vi "Tatrocki_B_1.vi"   [LabVIEW 2020]
uses:
  <vilib>/Platform/TimedLoop/XDataNode/timing_clust.ctl
  <vilib>/Platform/TimedLoop/XDataNode/nitl_modes.ctl
  <vilib>/Platform/TimedLoop/XDataNode/wakeup.ctl
  <vilib>/platform/TimedLoop/XDataNode/XDataNode.xnode
  <vilib>/Platform/TimedLoop/XDataNode/XDNodeRunTimeDep.lvlib
types:
  T1 = typedef "Rendezvous RefNum" = refnum<k1>
  T2 = typedef "Semaphore RefNum" = refnum<k1>
  T3 = typedef "XDNodeRunTimeDep.lvlib/timing_clust.ctl" = cluster{"Expected End [f-1]":u64, "Actual End [f-1]":u64, "Finished Late? [f-1]":bool, "Expected End [i-1]":u64, "Actual End [i-1]":u64, "Finished Late? [i-1]":bool, "Expected Start [i]":u64, "Actual Start [i]":u64, "Expected Start [f]":u64, "Actual Start [f]":u64, "Source Name":string, "Structure Name":string, "Period":i64, "Deadline":i64, "Offset":i64, "Start":i64, "Priority":i32, "Timeout":i32, "Mode":T4, "Wakeup Reason":T5, "Error":errorcluster, "Source Type":string, "Secondary Source Type":string, "Global End Time":u64, "Global Start Time":u64, "Frame Duration":u64, "Iteration Duration":u64, "Assigned CPU":i32, "I/O Scan Engine Mode":u32}
  T4 = typedef "XDNodeRunTimeDep.lvlib/nitl_modes.ctl" = enum32{"No Change", "Process missed periods, maintain original phase", "Discard missed periods, maintain original phase", "Process missed periods, ignore original phase", "Discard missed periods, ignore original phase"}
  T5 = typedef "XDNodeRunTimeDep.lvlib/wakeup.ctl" = enum32{"Normal", "Aborted", "Asynchronous wakeup", "Timing source error", "Timed loop error", "Timeout"}
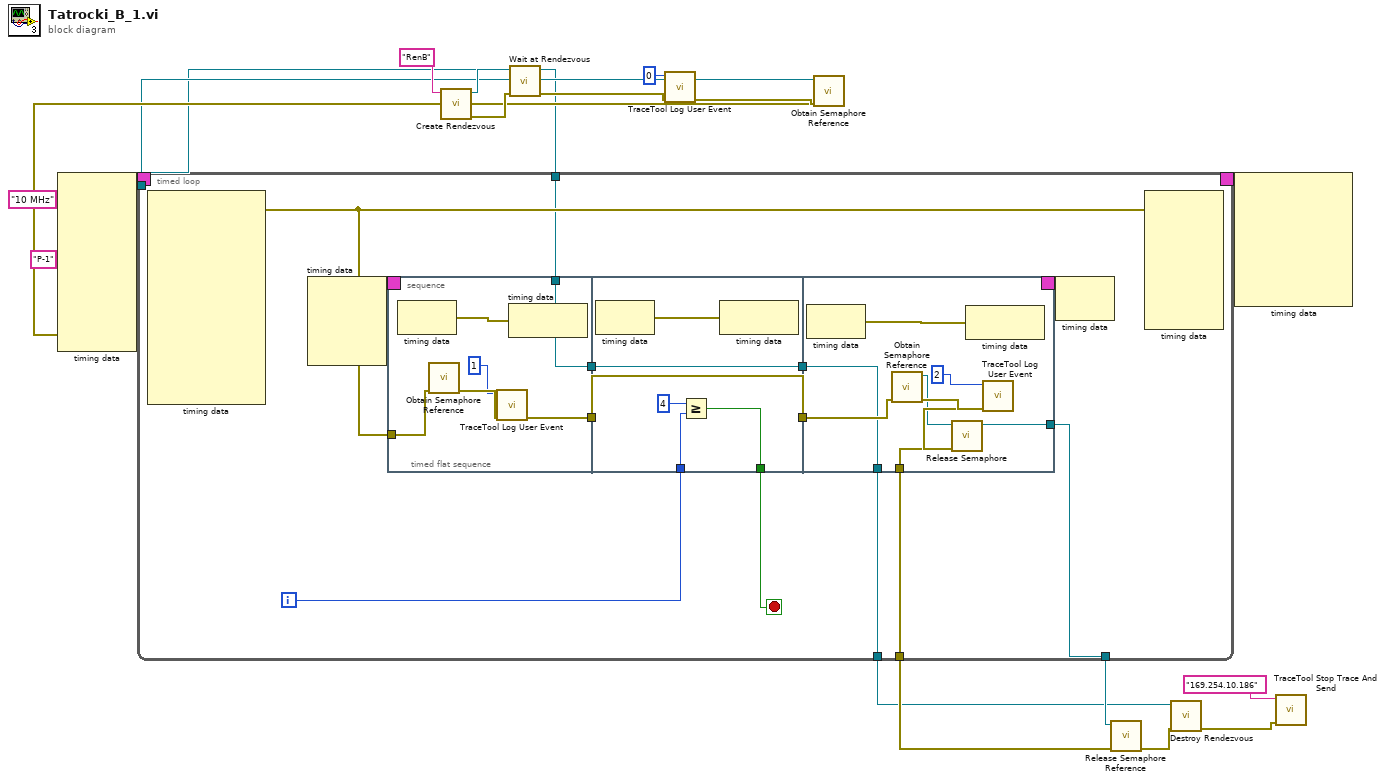
[diagram p0: block diagram]
diagram:
  n1 = call <vilib>:"Create Rendezvous.vi"("name (unnamed)"="RenB") -> ("error out"=w16:errorcluster, "rendezvous"=w18:T1)  [unwired: 4 in, 1 out]
  n2 = call <vilib>:"Wait at Rendezvous.vi"("error in (no error)"=w16, "rendezvous"=w18) -> ("error out"=w15:errorcluster, "rendezvous out"=w1:T1)  [unwired: 3 in, 1 out]
  n3 = call <vilib>:"TraceTool Log User Event.vi"("error in (no error)"=w15, "Event ID (0-255)"=u32 0) -> ("error out"=w14:errorcluster)  [unwired: 9 in]
  n4 = call <vilib>:"Obtain Semaphore Reference.vi"("error in (no error)"=w14) -> ("error out"=w9:errorcluster, "semaphore"=w6:T2)  [unwired: 4 in, 1 out]
  n5 = node-c288("10 MHz" ("Source Name"), "P-1" ("Structure Name"), w9) -> (w13:T3)  [unwired: 7 in]
  n6 = timed-loop {
    timing: w13 -> [_]
    timing-out: [_] -> w12
    tunnel: [w23] -> w8
    tunnel: [w22] -> w7
    tunnel: w1 -> [_]
    tunnel: w6 -> [_]
    tunnel: [w21] -> w2
    tunnel: w1 -> [w20]
    i -> [w25]
    stop <- w24 stop-if-true
    n7 = node-c288() -> (w26:errorcluster)  [unwired: 1 in, 12 out]
    n8 = node-c288() -> (w28:T3)  [unwired: 4 in]
    n9 = timed-sequence {
      timing: w28 -> [_]
      timing-out: [_] -> w27
      tunnel: w26 -> [w39]
      tunnel: w25 -> [w38]
      tunnel: [w37] -> w24
      tunnel: [w34] -> w23
      tunnel: [w33] -> w22
      tunnel: [w32] -> w21
      tunnel: w20 -> [w29]
      n10 = timed-flat-sequence {
        tunnel: w39 -> [w44]
        tunnel: [w41] -> w35
        tunnel: [w40] -> w30
        tunnel: w29 -> [w40]
        tunnel: w38 -> [w55]
        tunnel: [w54] -> w37
        tunnel: [w53] -> w36
        tunnel: w35 -> [w53]
        tunnel: [w51] -> w31
        tunnel: w30 -> [w51]
        tunnel: w36 -> [w67]
        tunnel: [w65] -> w34
        tunnel: [w63] -> w33
        tunnel: [w62] -> w32
        tunnel: w31 -> [w62]
        frame #0 {
          n11 = node-c288() -> (w45:errorcluster)  [unwired: 1 in]
          n12 = call <vilib>:"Obtain Semaphore Reference.vi"("error in (no error)"=w44) -> ("error out"=w43:errorcluster)  [unwired: 4 in, 2 out]
          n13 = call <vilib>:"TraceTool Log User Event.vi"("error in (no error)"=w43, "Event ID (0-255)"=u32 1) -> ("error out"=w41:errorcluster)  [unwired: 9 in]
          n14 = node-c288(w45) -> ()  [unwired: 1 out]
        }
        frame #1 {
          n15 = node-c288() -> (w56:errorcluster)  [unwired: 1 in]
          n16 = Greater Or Equal?(x=4, y=w55) -> (x >= y?=w54:bool)
          n17 = node-c288(w56) -> ()  [unwired: 1 out]
        }
        frame #2 {
          n18 = node-c288() -> (w70:errorcluster)  [unwired: 1 in]
          n19 = call <vilib>:"Obtain Semaphore Reference.vi"("error in (no error)"=w67) -> ("error out"=w69:errorcluster, "semaphore"=w64:T2)  [unwired: 4 in, 1 out]
          n20 = node-c288(w70) -> ()  [unwired: 1 out]
          n21 = call <vilib>:"TraceTool Log User Event.vi"("error in (no error)"=w69, "Event ID (0-255)"=u32 2) -> ("error out"=w66:errorcluster)  [unwired: 9 in]
          n22 = call <vilib>:"Release Semaphore.vi"("error in (no error)"=w66, "semaphore"=w64) -> ("error out"=w65:errorcluster, "semaphore out"=w63:T2)  [unwired: 4 in]
        }
      }
    }
    n23 = node-c288(w27) -> ()  [unwired: 1 out]
    n24 = node-c288(w26) -> ()  [unwired: 7 in, 1 out]
  }
  n25 = call <vilib>:"Release Semaphore Reference.vi"("error in (no error)"=w8, "semaphore"=w7) -> ("error out"=w5:errorcluster)  [unwired: 8 in, 1 out]
  n26 = call <vilib>:"Destroy Rendezvous.vi"("error in (no error)"=w5, "rendezvous"=w2) -> ("error out"=w4:errorcluster)  [unwired: 4 in, 1 out]
  n27 = node-c288(w12) -> ()  [unwired: 7 out]
  n28 = call <vilib>:"TraceTool Stop Trace And Send.vi"("error in (no error)"=w4, "Trace Host Network Address"="169.254.10.186") -> ()  [unwired: 9 in, 1 out]
